vi "TurnSlow.vi"(8 "b - value":dbl, 9 "Scale Factor":dbl, 10 "Deadband X value":dbl, 11 "Input Twist":dbl) -> (3 "Twist Output":dbl)   [LabVIEW 2017]
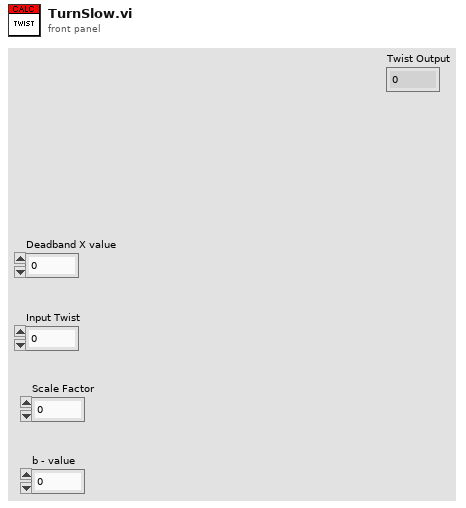
[diagram p1: front panel]
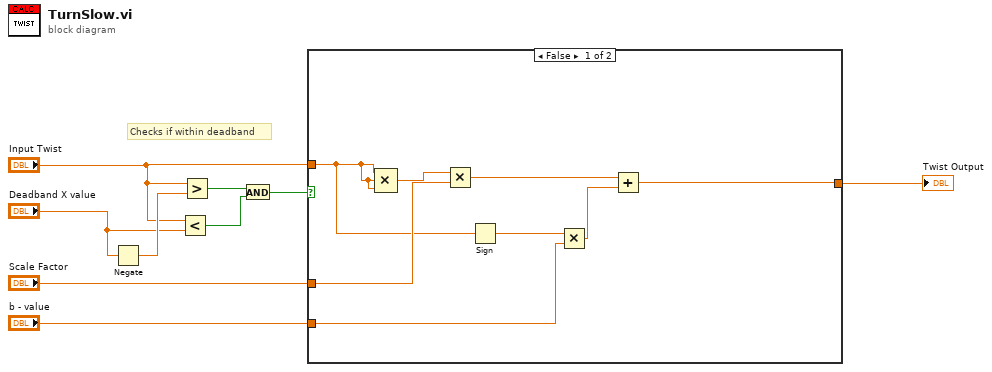
[diagram p0: block diagram]
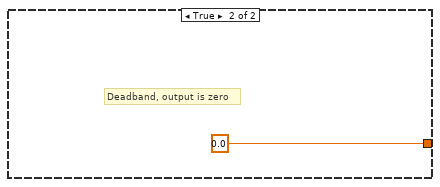
[diagram p2: hidden frame]
diagram:
  # "Checks if within deadband"
  n1 = Negate(x="Deadband X value") -> (-x=w6:dbl)
  n2 = Less?(x="Input Twist", y="Deadband X value") -> (x < y?=w7:bool)
  n3 = Greater?(x="Input Twist", y=w6) -> (0:w8:bool)
  n4 = And(x=w8, y=w7) -> (x .and. y?=w9:bool)
  n5 = case shown="False" w9 {
    tunnel: "Input Twist" -> [w10 _]
    tunnel: "Scale Factor" -> [w17 _]
    tunnel: "b - value" -> [w15 _]
    tunnel: [w12 0.0] -> w1
    frame False {
      n6 = Compound Arithmetic op=MULTIPLY(w10, w10, w10) -> (w11:dbl)
      n7 = Multiply(x=w11, y=w17) -> (x*y=w16:dbl)
      n8 = Sign(1:w10) -> (0:w13:dbl)
      n9 = Multiply(x=w13, y=w15) -> (x*y=w14:dbl)
      n10 = Add(x=w16, y=w14) -> (x+y=w12:dbl)
    }
    frame True {
      # "Deadband, output is zero"
    }
  }
  "Twist Output" <- w1
